vi "Core Actor - DISPLAY - Message (String).vi"(8 "error in (no error)":errorcluster, 9 "Value":string, 11 "Child_1_Class in":refnum<class "GUI_Class.lvclass">) -> (0 "error out":errorcluster, 3 "Child_1_Class out":refnum<class "GUI_Class.lvclass">)   [LabVIEW 2023, in "GUI_Actor.lvlib" / "GUI_Class.lvclass"]
uses:
  GUI_Class.lvclass
  GUI_Class.lvclass/GUI_Class.ctl
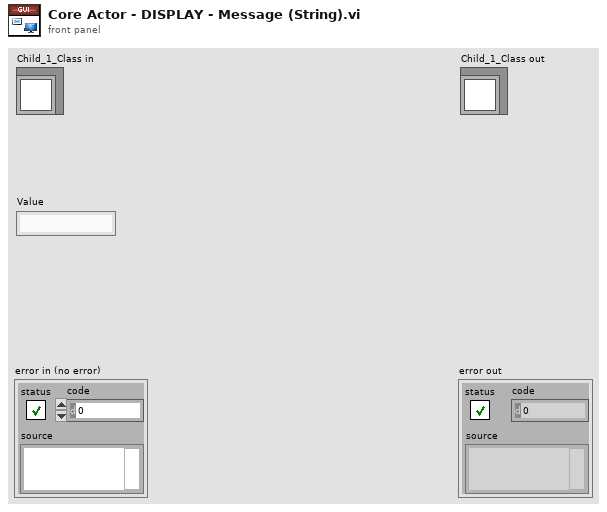
[diagram p1: front panel]
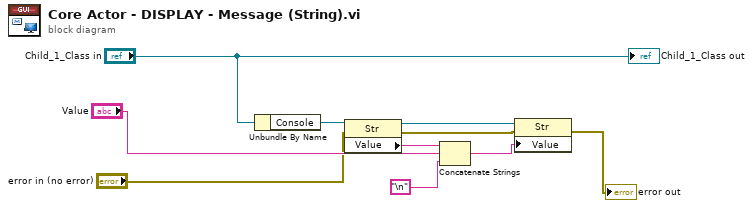
[diagram p0: block diagram]
diagram:
  n1 = Unbundle By Name("Child_1_Class in") -> ("Console"=w10:refnum<vi>)
  n2 = property class="Str"(reference=w10, error in="error in (no error)") -> (reference out=w8:refnum<vi>, error out=w7:errorcluster, "Value"=w9:string)
  n3 = Concatenate Strings(w9, "Value", "\n") -> (w6:string)
  n4 = property class="Str"(reference=w8, error in=w7, "Value"=w6) -> (error out=→"error out":errorcluster)  [unwired: 1 out]
  "Child_1_Class out" <- "Child_1_Class in"
